vi "StringConcatenate.vi"() -> ()   [LabVIEW 2019]
panel:
  out "String3":string
  in  "String2":string="World"
  in  "String1":string="Hello"
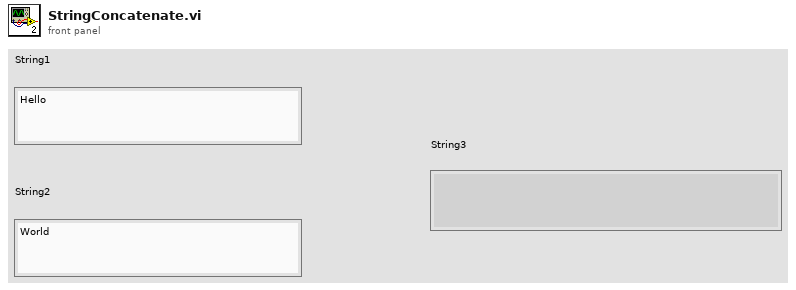
[diagram p1: front panel]
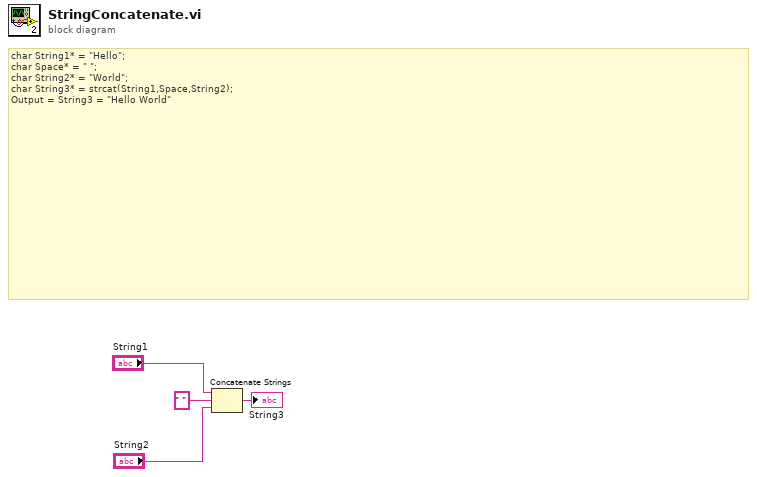
[diagram p0: block diagram]
diagram:
  # "char String1* = \"Hello\";\nchar Space* = \" \";\nchar String2* = \"World\";\nchar String3* = strcat(String1,Space,String2);\nOutput = String3 = \"Hello World\""
  n1 = Concatenate Strings("String1", " " ("string"), "String2") -> (→"String3":string)
